vi "Login Authority CSV FGV.vi"(7 "Command":T2, 8 "error in (no error)":errorcluster, 9 "Data In":T1, 10 "Authority":string, 11 "Path":path) -> (0 "error out":errorcluster, 1 "Data Out":T1, 2 "Authorities":string[](array[string]))   [LabVIEW 2017]
uses:
  Controls/Login Authority CSV FGV Command.ctl
  <vilib>/Utility/file.llb/Write To Spreadsheet File (string).vi
  <vilib>/Utility/file.llb/Read From Spreadsheet File (string).vi
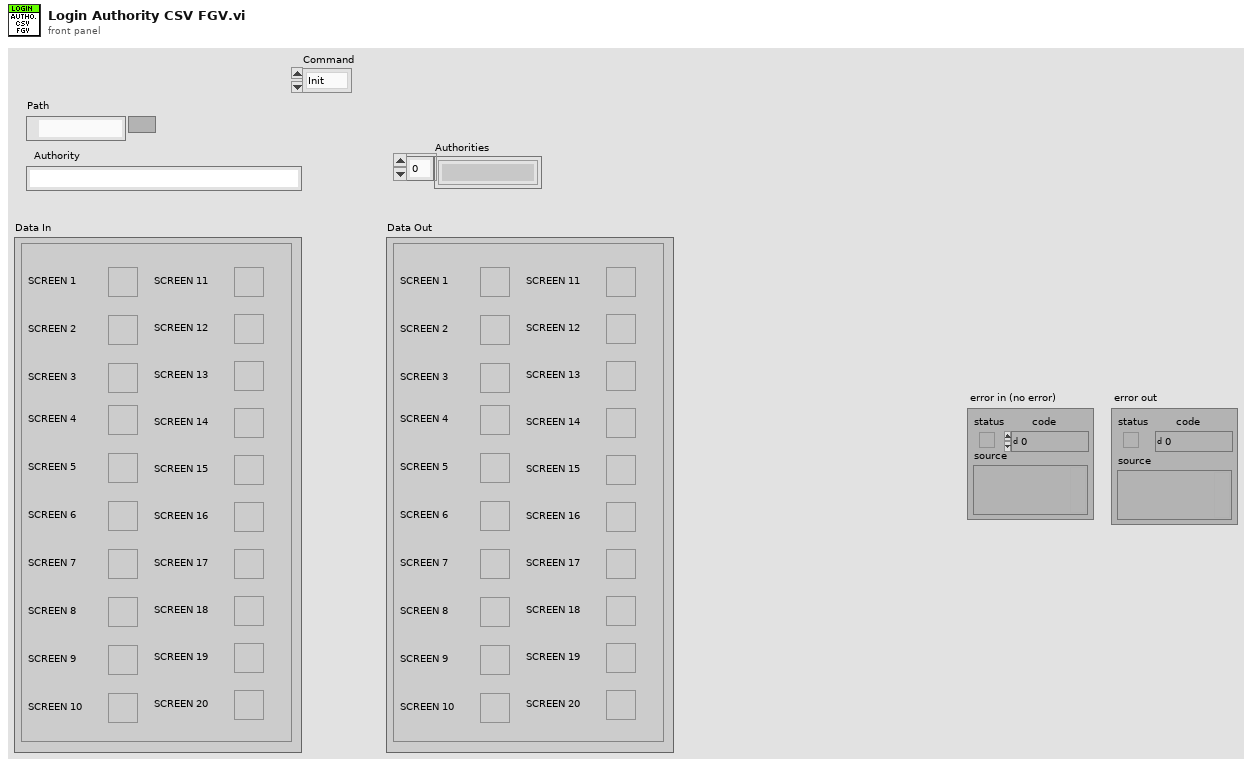
[diagram p1: front panel]
types:
  T1 = cluster{"SCREEN 1":bool, "SCREEN 2":bool, "SCREEN 3":bool, "SCREEN 4":bool, "SCREEN 5":bool, "SCREEN 6":bool, "SCREEN 7":bool, "SCREEN 8":bool, "SCREEN 9":bool, "SCREEN 10":bool, "SCREEN 11":bool, "SCREEN 12":bool, "SCREEN 13":bool, "SCREEN 14":bool, "SCREEN 15":bool, "SCREEN 16":bool, "SCREEN 17":bool, "SCREEN 18":bool, "SCREEN 19":bool, "SCREEN 20":bool}
  T2 = typedef "Login Authority CSV FGV Command.ctl" = enum16{"Init", "Save", "Read", "Get Data", "Delete"}
  T3 = cluster{"[0]":bool, "[1]":bool, "[2]":bool, "[3]":bool, "[4]":bool, "[5]":bool, "[6]":bool, "[7]":bool, "[8]":bool, "[9]":bool, "[10]":bool, "[11]":bool, "[12]":bool, "[13]":bool, "[14]":bool, "[15]":bool, "[16]":bool, "[17]":bool, "[18]":bool, "[19]":bool}
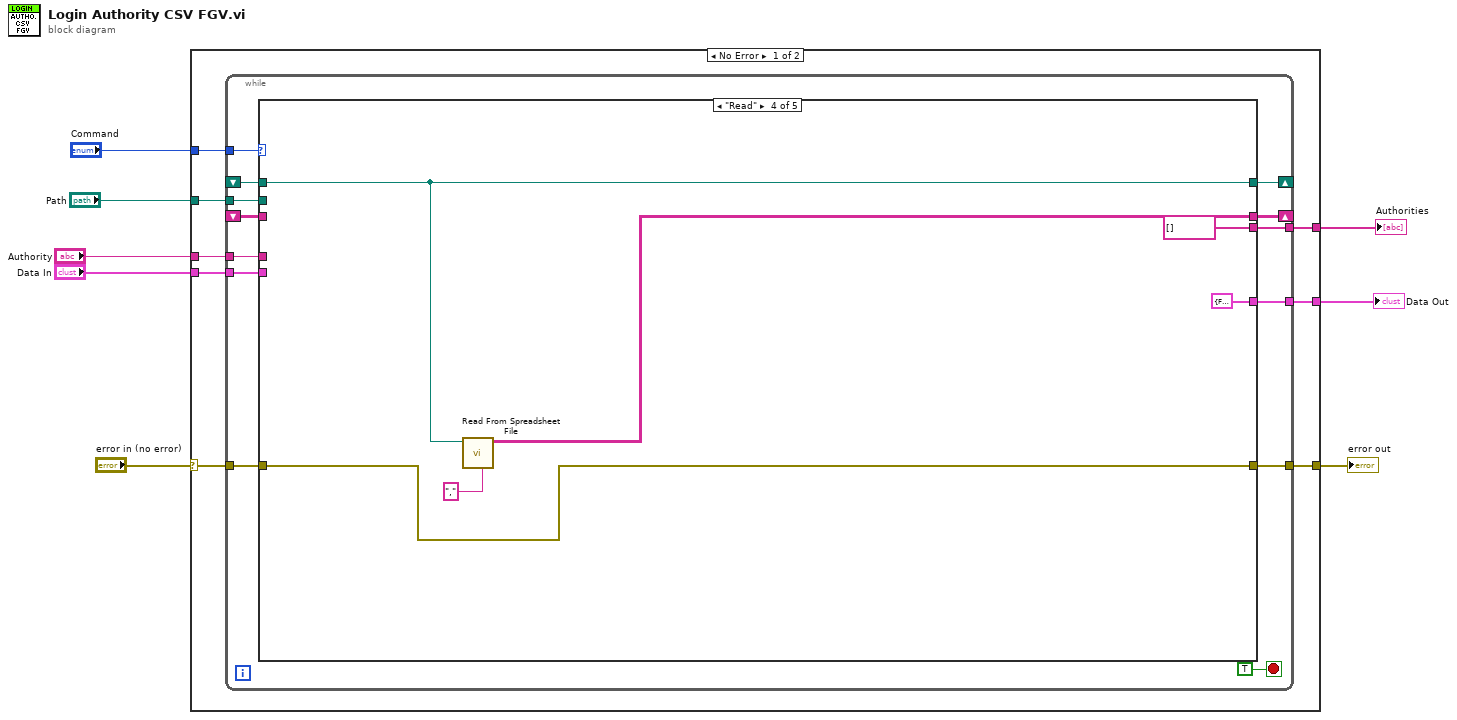
[diagram p0: block diagram]
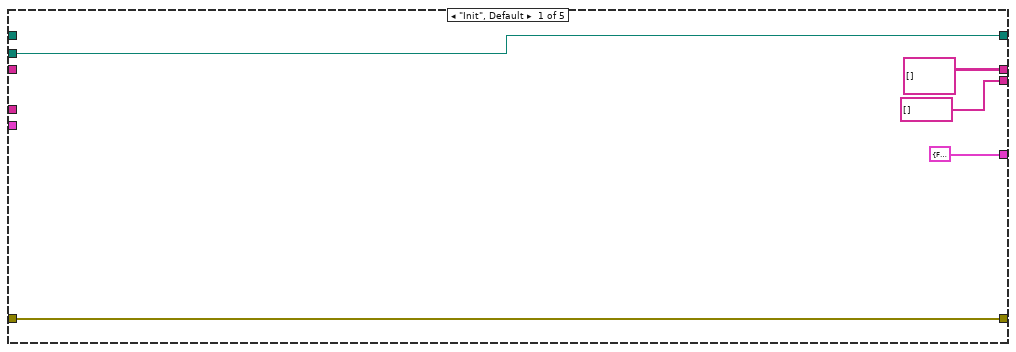
[diagram p2: hidden frame]
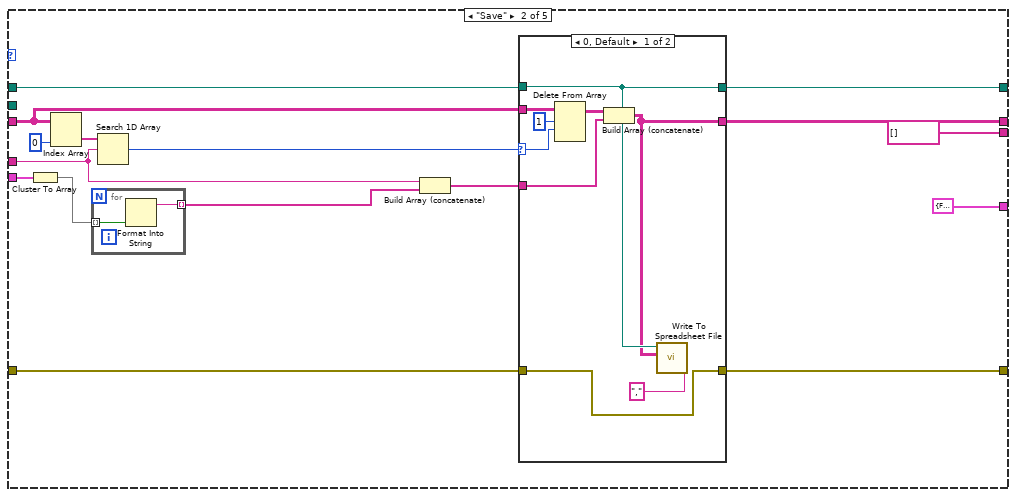
[diagram p3: hidden frame]
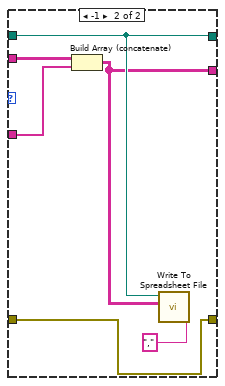
[diagram p4: hidden frame]
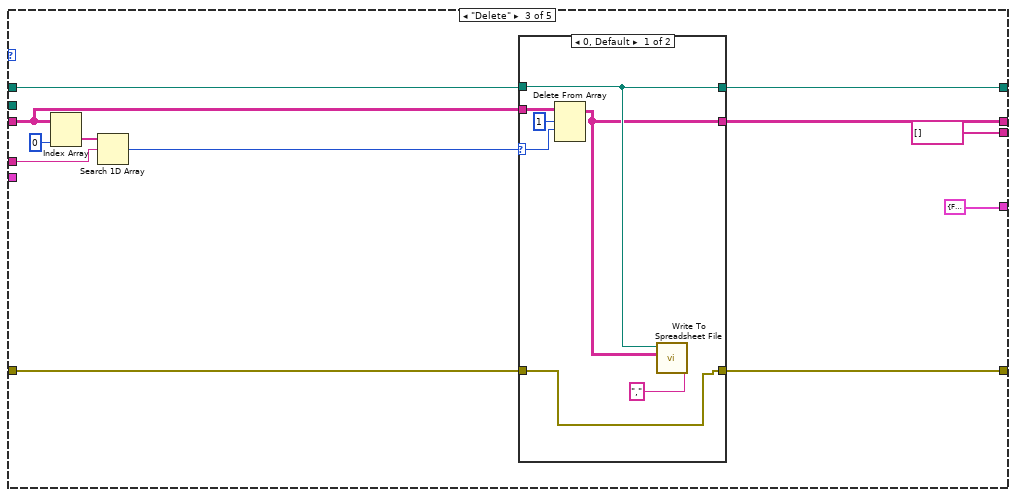
[diagram p5: hidden frame]
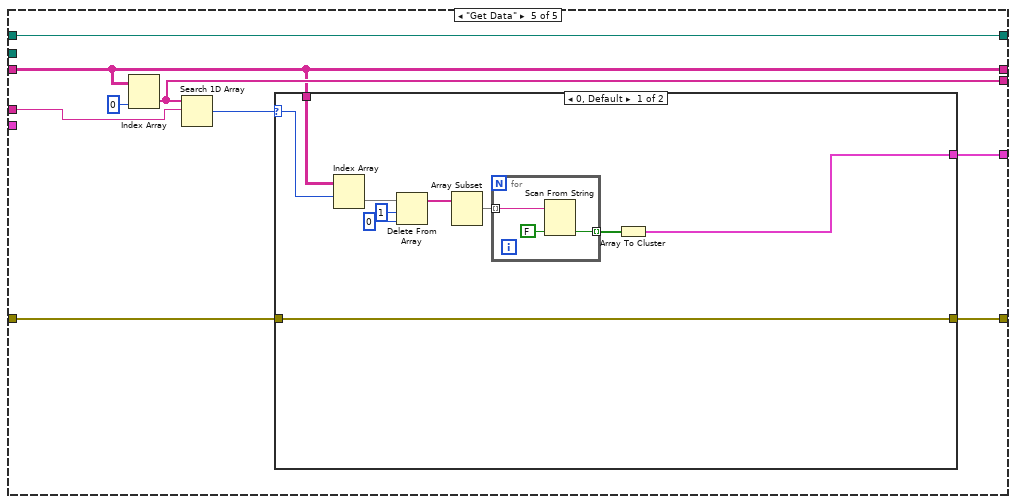
[diagram p7: hidden frame]
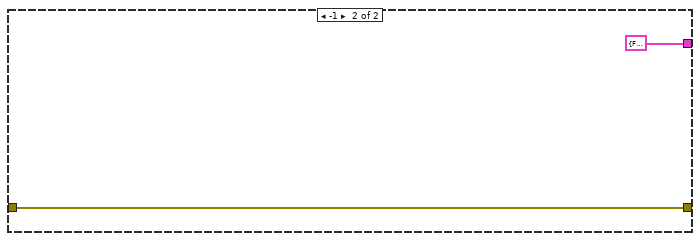
[diagram p8: hidden frame]
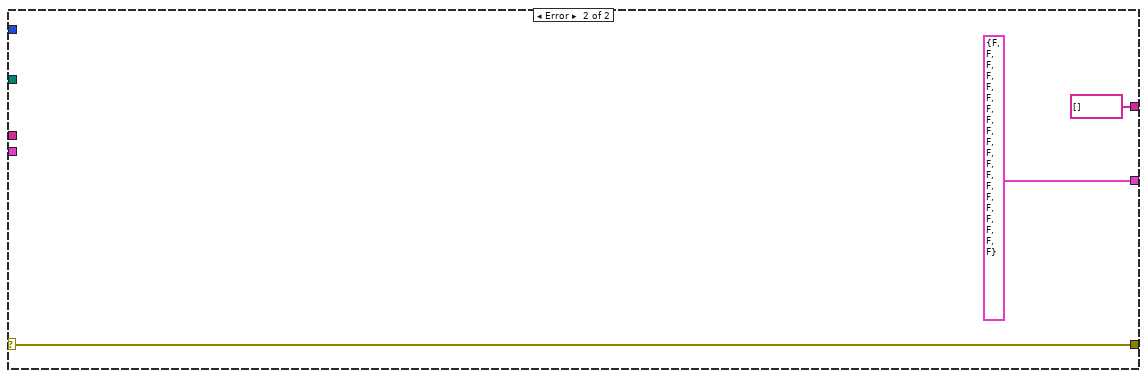
[diagram p9: hidden frame]
diagram:
  n1 = case shown="No Error" "error in (no error)" {
    selector: "error in (no error)" -> [w16 w122]
    tunnel: [w15 w122] -> w7
    tunnel: "Command" -> [w14 _]
    tunnel: "Path" -> [w10 _]
    tunnel: [w9 T1 {"SCREEN 1"=FALSE, "SCREEN 2"=FALSE, "SCREEN 3"=FALSE, "SCREEN 4"=FALSE, "SCREEN 5"=FALSE, "SCREEN 6"=FALSE, "SCREEN 7"=FALSE, "SCREEN 8"=FALSE, "SCREEN 9"=FALSE, "SCREEN 10"=FALSE, "SCREEN 11"=FALSE, "SCREEN 12"=FALSE, "SCREEN 13"=FALSE, "SCREEN 14"=FALSE, "SCREEN 15"=FALSE, "SCREEN 16"=FALSE, "SCREEN 17"=FALSE, "SCREEN 18"=FALSE, "SCREEN 19"=FALSE, "SCREEN 20"=FALSE} ("Data Out")] -> w1
    tunnel: "Authority" -> [w13 _]
    tunnel: "Data In" -> [w12 _]
    tunnel: [w11 string[] [] ("all rows")] -> w3
    frame No Error {
      n2 = while {
        tunnel: w16 -> [w28]
        tunnel: [w27] -> w15
        tunnel: w14 -> [w26]
        shift-right: [w25] -> _
        shift-left: _ -> [w24]
        tunnel: w13 -> [w23]
        tunnel: w12 -> [w22]
        shift-right: [w18] -> _
        shift-left: _ -> [w21]
        tunnel: [w20] -> w11
        tunnel: w10 -> [w19]
        tunnel: [w17] -> w9
        stop <- TRUE stop-if-true
        n3 = case shown="\"Read\"" w26 {
          tunnel: w28 -> [w34 w40 w75 w91 w100]
          tunnel: [w34 w46 w72 w91 w99] -> w27
          tunnel: [w33 w44 w73 w94 w104] -> w25
          tunnel: w24 -> [_ w45 w74 w94 w104]
          tunnel: w23 -> [_ w38 w77 _ w102]
          tunnel: w22 -> [_ w39 _ _ _]
          tunnel: [string[][] [] w47 w70 w90 w97] -> w18
          tunnel: w21 -> [_ w48 w76 _ w97]
          tunnel: [string[] [] ("all rows") string[] [] ("all rows") string[] [] ("all rows") string[] [] ("all rows") w101] -> w20
          tunnel: w19 -> [w33 _ _ _ _]
          tunnel: [T1 {"SCREEN 1"=FALSE, "SCREEN 2"=FALSE, "SCREEN 3"=FALSE, "SCREEN 4"=FALSE, "SCREEN 5"=FALSE, "SCREEN 6"=FALSE, "SCREEN 7"=FALSE, "SCREEN 8"=FALSE, "SCREEN 9"=FALSE, "SCREEN 10"=FALSE, "SCREEN 11"=FALSE, "SCREEN 12"=FALSE, "SCREEN 13"=FALSE, "SCREEN 14"=FALSE, "SCREEN 15"=FALSE, "SCREEN 16"=FALSE, "SCREEN 17"=FALSE, "SCREEN 18"=FALSE, "SCREEN 19"=FALSE, "SCREEN 20"=FALSE} ("Data Out") T1 {"SCREEN 1"=FALSE, "SCREEN 2"=FALSE, "SCREEN 3"=FALSE, "SCREEN 4"=FALSE, "SCREEN 5"=FALSE, "SCREEN 6"=FALSE, "SCREEN 7"=FALSE, "SCREEN 8"=FALSE, "SCREEN 9"=FALSE, "SCREEN 10"=FALSE, "SCREEN 11"=FALSE, "SCREEN 12"=FALSE, "SCREEN 13"=FALSE, "SCREEN 14"=FALSE, "SCREEN 15"=FALSE, "SCREEN 16"=FALSE, "SCREEN 17"=FALSE, "SCREEN 18"=FALSE, "SCREEN 19"=FALSE, "SCREEN 20"=FALSE} ("Data Out") T1 {"SCREEN 1"=FALSE, "SCREEN 2"=FALSE, "SCREEN 3"=FALSE, "SCREEN 4"=FALSE, "SCREEN 5"=FALSE, "SCREEN 6"=FALSE, "SCREEN 7"=FALSE, "SCREEN 8"=FALSE, "SCREEN 9"=FALSE, "SCREEN 10"=FALSE, "SCREEN 11"=FALSE, "SCREEN 12"=FALSE, "SCREEN 13"=FALSE, "SCREEN 14"=FALSE, "SCREEN 15"=FALSE, "SCREEN 16"=FALSE, "SCREEN 17"=FALSE, "SCREEN 18"=FALSE, "SCREEN 19"=FALSE, "SCREEN 20"=FALSE} ("Data Out") T1 {"SCREEN 1"=FALSE, "SCREEN 2"=FALSE, "SCREEN 3"=FALSE, "SCREEN 4"=FALSE, "SCREEN 5"=FALSE, "SCREEN 6"=FALSE, "SCREEN 7"=FALSE, "SCREEN 8"=FALSE, "SCREEN 9"=FALSE, "SCREEN 10"=FALSE, "SCREEN 11"=FALSE, "SCREEN 12"=FALSE, "SCREEN 13"=FALSE, "SCREEN 14"=FALSE, "SCREEN 15"=FALSE, "SCREEN 16"=FALSE, "SCREEN 17"=FALSE, "SCREEN 18"=FALSE, "SCREEN 19"=FALSE, "SCREEN 20"=FALSE} ("Data Out") w96] -> w17
          frame "Init", Default {
          }
          frame "Save" {
            n4 = Cluster To Array(cluster=w39) -> (array=w37:bool[])
            n5 = Index Array(array=w48, index (col)=0 ("disabled index (col)")) -> (element=w43:string[])  [unwired: 1 in]
            n6 = for {
              tunnel: w37 -> [w52] mode=indexing
              tunnel: [w51] -> w36 mode=indexing
              n7 = Format Into String(w52) -> (resulting string=w51:string)  [unwired: 3 in, 1 out]
            }
            n8 = Search 1D Array(1D array=w43, element=w38) -> (index of element=w49:i32)  [unwired: 1 in]
            n9 = Build Array (concatenate)(w38, w36) -> (w41:string[])
            n10 = case shown="0, Default" w49 {
              selector: w49 -> [w57 _]
              tunnel: w48 -> [w61 w67]
              tunnel: [w53 w62] -> w47
              tunnel: [w54 w63] -> w46
              tunnel: w45 -> [w58 w65]
              tunnel: [w58 w65] -> w44
              tunnel: w41 -> [w55 w64]
              tunnel: w40 -> [w54 w63]
              frame 0, Default {
                n11 = Delete From Array(array=w61, length=1, index (row)=w57) -> (array with subset deleted=w60:string[][])  [unwired: 1 in, 1 out]
                n12 = Build Array (concatenate)(w60, w55) -> (w53:string[][])
                n13 = call-poly <vilib>:"Write To Spreadsheet File.vi"("delimiter (\\t)"="," ("delimiter (\\t)"), "2D data"=w53, "file path (dialog if empty)"=w58) -> ()  [unwired: 5 in, 1 out]
              }
              frame -1 {
                n14 = Build Array (concatenate)(w67, w64) -> (w62:string[][])
                n15 = call-poly <vilib>:"Write To Spreadsheet File.vi"("delimiter (\\t)"="," ("delimiter (\\t)"), "2D data"=w62, "file path (dialog if empty)"=w65) -> ()  [unwired: 5 in, 1 out]
              }
            }
          }
          frame "Delete" {
            n16 = Index Array(array=w76, index (col)=0 ("disabled index (col)")) -> (element=w69:string[])  [unwired: 1 in]
            n17 = Search 1D Array(1D array=w69, element=w77) -> (index of element=w78:i32)  [unwired: 1 in]
            n18 = case shown="0, Default" w78 {
              selector: w78 -> [w82 _]
              tunnel: w76 -> [w86 w88]
              tunnel: [w80 w88] -> w70
              tunnel: w75 -> [w81 w87]
              tunnel: w74 -> [w84 w89]
              tunnel: [w84 w89] -> w73
              tunnel: [w81 w87] -> w72
              frame 0, Default {
                n19 = Delete From Array(array=w86, length=1, index (row)=w82) -> (array with subset deleted=w80:string[][])  [unwired: 1 in, 1 out]
                n20 = call-poly <vilib>:"Write To Spreadsheet File.vi"("delimiter (\\t)"="," ("delimiter (\\t)"), "2D data"=w80, "file path (dialog if empty)"=w84) -> ()  [unwired: 5 in, 1 out]
              }
              frame -1 {
              }
            }
          }
          frame "Read" {
            n21 = call-poly <vilib>:"Read From Spreadsheet File.vi"("delimiter (\\t)"="," ("delimiter (\\t)"), "file path (dialog if empty)"=w94) -> ("all rows"=w90:string[][])  [unwired: 5 in, 4 out]
          }
          frame "Get Data" {
            n22 = Index Array(array=w97, index (col)=0 ("disabled index (col)")) -> (element=w101:string[])  [unwired: 1 in]
            n23 = Search 1D Array(1D array=w101, element=w102) -> (index of element=w98:i32)  [unwired: 1 in]
            n24 = case shown="0, Default" w98 {
              selector: w98 -> [w113 _]
              tunnel: w100 -> [w108 w119]
              tunnel: [w108 w119] -> w99
              tunnel: w97 -> [w114 _]
              tunnel: [w105 T1 {"SCREEN 1"=FALSE, "SCREEN 2"=FALSE, "SCREEN 3"=FALSE, "SCREEN 4"=FALSE, "SCREEN 5"=FALSE, "SCREEN 6"=FALSE, "SCREEN 7"=FALSE, "SCREEN 8"=FALSE, "SCREEN 9"=FALSE, "SCREEN 10"=FALSE, "SCREEN 11"=FALSE, "SCREEN 12"=FALSE, "SCREEN 13"=FALSE, "SCREEN 14"=FALSE, "SCREEN 15"=FALSE, "SCREEN 16"=FALSE, "SCREEN 17"=FALSE, "SCREEN 18"=FALSE, "SCREEN 19"=FALSE, "SCREEN 20"=FALSE} ("Data Out")] -> w96
              frame 0, Default {
                n25 = Index Array(array=w114, index (row)=w113) -> (element=w112:string[])  [unwired: 1 in]
                n26 = Delete From Array(array=w112, length=1, index=0) -> (array with subset deleted=w109:string[])  [unwired: 1 out]
                n27 = Array Subset(array=w109) -> (w107:string[])  [unwired: 2 in]
                n28 = for {
                  tunnel: w107 -> [w117] mode=indexing
                  tunnel: [w115] -> w106 mode=indexing
                  n29 = Scan From String(input string=w117, default 1=FALSE) -> (output 1=w115:bool)  [unwired: 3 in, 3 out]
                }
                n30 = Array To Cluster(array=w106) -> (cluster=w105:T3)
              }
              frame -1 {
              }
            }
          }
        }
      }
    }
    frame Error {
    }
  }
  "error out" <- w7
  "Authorities" <- w3
  "Data Out" <- w1
